vi "cluster 1.vi"() -> ()   [LabVIEW 2018]
panel:
  out "Numeric":dbl format="%#_13g"
  out "Cluster 2":T1
  in  "Cluster":T1
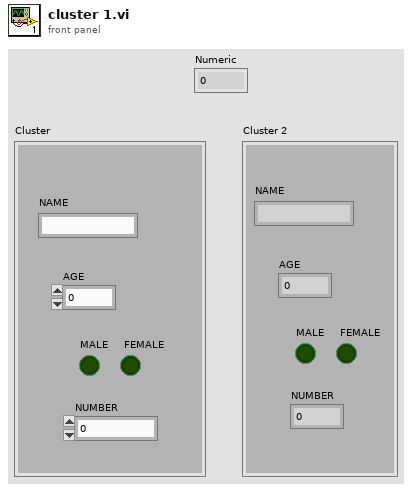
[diagram p1: front panel]
types:
  T1 = cluster{"NAME":string, "AGE":dbl, "MALE":bool, " FEMALE":bool, "NUMBER":dbl}
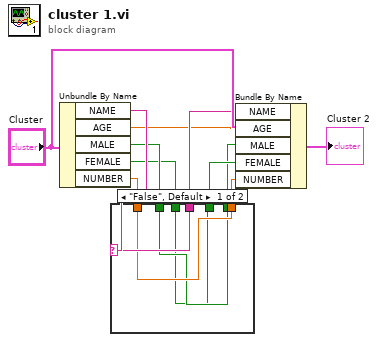
[diagram p0: block diagram]
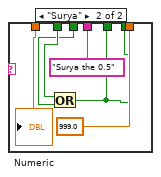
[diagram p2: hidden frame]
diagram:
  n1 = Unbundle By Name("Cluster") -> ("NAME"=w9:string, "AGE"=w3:dbl, "MALE"=w6:bool, "FEMALE"=w5:bool, "NUMBER"=w4:dbl)
  n2 = case shown="\"False\", Default" w9 {
    selector: w9 -> [w15 _]
    tunnel: [w15 "Surya the 0.5"] -> w8
    tunnel: [w13 w19] -> w1
    tunnel: [w14 999.0 ("Numeric")] -> w7
    tunnel: w4 -> [w14 w16]
    tunnel: w6 -> [w13 w18]
    tunnel: [w12 w19] -> w2
    tunnel: w5 -> [w12 w17]
    frame "False", Default {
    }
    frame "Surya" {
      n3 = Or(x=w18, y=w17) -> (x .or. y?=w19:bool)
      "Numeric" <- w16
    }
  }
  n4 = Bundle By Name(cluster="Cluster", "NAME"=w8, "AGE"=w3, "MALE"=w1, "FEMALE"=w2, "NUMBER"=w7) -> (→"Cluster 2":T1)
